vi "NiSwitch InitWithTopology.vi"(6 "contextId":T1, 8 "error in":errorcluster, 9 "timeout (ms)":i32=-1, 10 "Request Data":T4, 11 "gRPC ID":T1) -> (0 "error out":errorcluster, 2 "Response Data":T2, 3 "gRPC ID out":T1)   [LabVIEW 2021, in "NI Switch_client.lvlib"]
uses:
  NI Switch_client.lvlib
  <vilib>/gRPC/LabVIEW gRPC Library/Shared/grpcId.ctl
  RPC Messages/niswitch_grpc_InitWithTopologyRequest.ctl
  RPC Messages/nidevice_grpc_SessionInitializationBehavior.ctl
  RPC Messages/niswitch_grpc_InitWithTopologyResponse.ctl
  RPC Messages/nidevice_grpc_Session.ctl
  RPC Messages/niswitch_grpc_InitWithTopologyResponse_Flat.ctl
  RPC Messages/nidevice_grpc_Session_Flat.ctl
  14035477-4c25-4107-8ed5-d0c4ef420ce5.vi
  <vilib>/gRPC/LabVIEW gRPC Library/Shared/TranslateGrpcError.vi
  <vilib>/gRPC/LabVIEW gRPC Library/Shared/Wait On Occurrence Wrapper.vi
  RPC Messages/FlatToRichnidevice_grpc_Session.vi
  <vilib>/gRPC/LabVIEW gRPC Library/Shared/Wait On Occurence.vi
  <vilib>/gRPC/LabVIEW gRPC Library/Server API/Server/Get Server DLL Path.vi
  <vilib>/Utility/error.llb/Error Cluster From Error Code.vi
  <vilib>/Utility/config.llb/Open Config Data.vi
  <vilib>/Utility/config.llb/Write Key.vi
  <vilib>/Utility/config.llb/Write Key (Boolean).vi
  <vilib>/Utility/config.llb/Not A Config Data Refnum.vi
  <vilib>/Utility/config.llb/Read Key.vi
  <vilib>/Utility/config.llb/Read Key (Boolean).vi
  <vilib>/Utility/config.llb/Close Config Data.vi
  <vilib>/gRPC/LabVIEW gRPC Library/grpc-lvsupport-release.lvlib
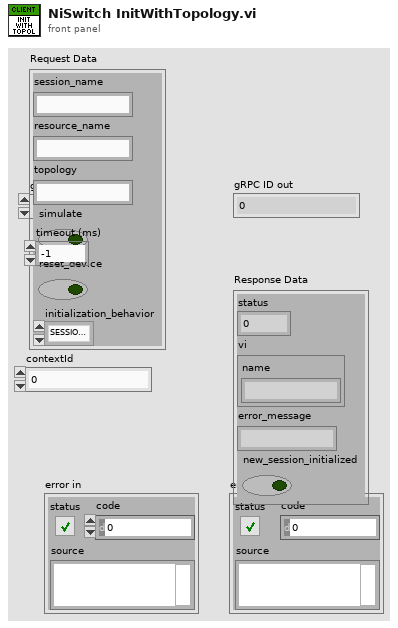
[diagram p1: front panel]
types:
  T1 = typedef "grpc-lvsupport-release.lvlib/grpcId.ctl" = u64
  T2 = typedef "NI Switch_client.lvlib/niswitch_grpc_InitWithTopologyResponse.ctl" = cluster{"status":i32, "vi":T3, "error_message":string, "new_session_initialized":bool}
  T3 = typedef "NI Switch_client.lvlib/nidevice_grpc_Session.ctl" = cluster{"name":string}
  T4 = typedef "NI Switch_client.lvlib/niswitch_grpc_InitWithTopologyRequest.ctl" = cluster{"session_name":string, "resource_name":string, "topology":string, "simulate":bool, "reset_device":bool, "initialization_behavior":T5}
  T5 = typedef "NI Switch_client.lvlib/nidevice_grpc_SessionInitializationBehavior.ctl" = enum32{"SESSION_INITIALIZATION_BEHAVIOR_UNSPECIFIED", "SESSION_INITIALIZATION_BEHAVIOR_INITIALIZE_NEW", "SESSION_INITIALIZATION_BEHAVIOR_ATTACH_TO_EXISTING"}
  T6 = typedef "NI Switch_client.lvlib/niswitch_grpc_InitWithTopologyResponse_Flat.ctl" = cluster{"status":i32, "vi":T7, "error_message":string, "new_session_initialized":bool}
  T7 = typedef "NI Switch_client.lvlib/nidevice_grpc_Session_Flat.ctl" = cluster{"name":string}
  T8 = typedef "NI Switch_client.lvlib/niswitch_grpc_InitWithTopologyRequest_Flat.ctl" = cluster{"session_name":string, "resource_name":string, "topology":string, "simulate":bool, "reset_device":bool, "initialization_behavior":T5}
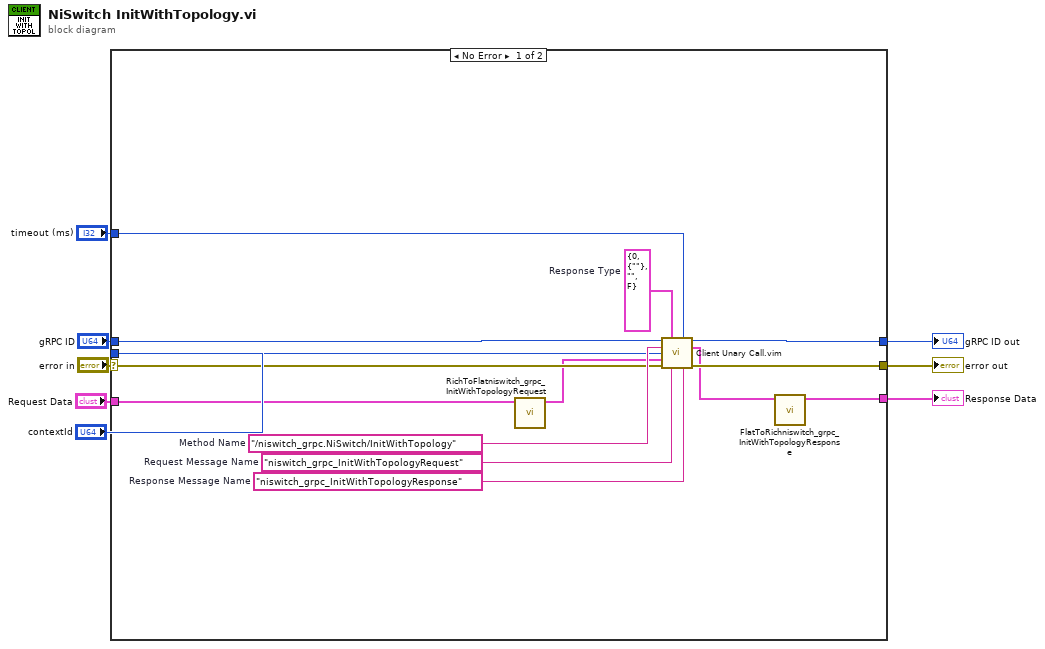
[diagram p0: block diagram]
diagram:
  n1 = case shown="No Error" "error in" {
    selector: "error in" -> [w18 w23]
    tunnel: [w17 w23] -> w7
    tunnel: "gRPC ID" -> [w16 w24]
    tunnel: [w15 w24] -> w5
    tunnel: "Request Data" -> [w12 _]
    tunnel: [w9 _] -> w3
    tunnel: "timeout (ms)" -> [w14 _]
    tunnel: "contextId" -> [w13 _]
    frame No Error {
      w19 = "niswitch_grpc_InitWithTopologyResponse"  # Response Message Name
      w20 = "niswitch_grpc_InitWithTopologyRequest"  # Request Message Name
      w21 = T6 {"status"=0, "vi"={"name"=""}, "error_message"="", "new_session_initialized"=FALSE}  # Response Type
      w22 = "/niswitch_grpc.NiSwitch/InitWithTopology"  # Method Name
      n2 = call "RichToFlatniswitch_grpc_InitWithTopologyRequest.vi"("InputCluster"=w12) -> ("OutputCluster"=w11:T8)  [unwired: 10 in]
      n3 = call "Client Unary Call.vim"("ClientID in"=w16, "Response Type"=w21, "timeout (ms)"=w14, "Method Name"=w22, "contextId"=w13, "Request Data"=w11, "error in"=w18, "Request Message Name"=w20, "Response Message Name"=w19) -> ("ClientID out"=w15:u64, "Response Data"=w10:T6, "error out"=w17:errorcluster)  [unwired: 4 in]
      n4 = call "FlatToRichniswitch_grpc_InitWithTopologyResponse.vi"("InputCluster"=w10) -> ("OutputCluster"=w9:T2)  [unwired: 10 in]
    }
    frame Error {
    }
  }
  "error out" <- w7
  "gRPC ID out" <- w5
  "Response Data" <- w3
